vi "Ignore error from the list.vi"(0 "error codes to ignore":i32[](array[numeric]), 2 "error in (no error)":errorcluster) -> (1 "error out":errorcluster)   [LabVIEW 2020]
uses:
  a96de2c3-b1f9-46bc-8751-df0aa1b4eda5.vi
  <vilib>/Comparison/Equal/Equal Functor/Equal Functor.lvclass
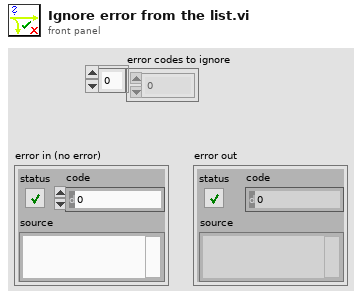
[diagram p1: front panel]
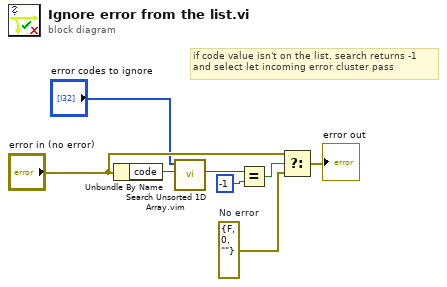
[diagram p0: block diagram]
diagram:
  w7 = errorcluster {"status"=FALSE, "code"=0, "source"=""}  # No error
  # "if code value isn't on the list, search returns -1 \nand select let incoming error cluster pass"
  n1 = Unbundle By Name("error in (no error)") -> ("code"=w2:i32)
  n2 = call "Search Unsorted 1D Array.vim"("element"=w2, "unsorted 1D array"="error codes to ignore") -> ("index of element"=w5:i32)  [unwired: 9 in]
  n3 = Equal?(x=w5, y=-1) -> (x = y?=w6:bool)
  n4 = Select(t="error in (no error)", s=w6, f=w7) -> (s? t:f=→"error out":errorcluster)
